vi "Create Line Seg.vi"(6 "Number of Points":i32=100, 7 "Y 2":dbl(slide) scale=0.0..10.0, 8 "X 2":dbl(slide) scale=0.0..10.0, 9 "Y 1":dbl(slide) scale=0.0..10.0, 10 "X 1":dbl(slide) scale=0.0..10.0) -> (3 "Line Segment":cluster{dbl[], dbl[]}(graph))   [LabVIEW 2013]
uses:
  <vilib>/Analysis/NI_AALPro.lvlib
panel:
  out "Plot With Point Markers":cluster{dbl[], dbl[]}[](graph)
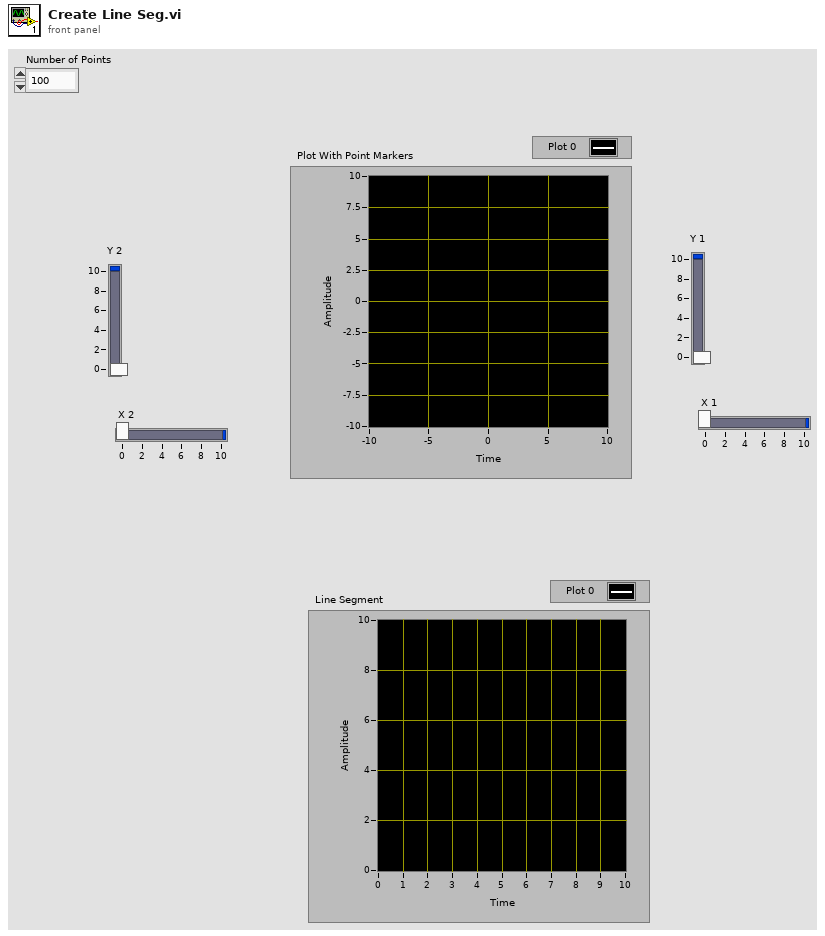
[diagram p1: front panel]
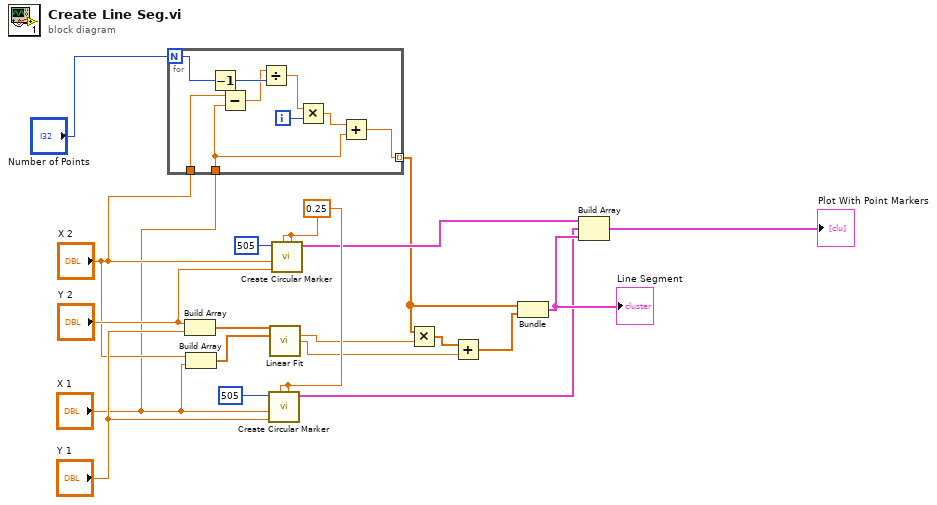
[diagram p0: block diagram]
diagram:
  w18 = 0.25 ("X Radius")
  n1 = for {
    N: "Number of Points" -> [w28]
    tunnel: [w23] -> w9 mode=indexing
    tunnel: "X 2" -> [w24]
    tunnel: "X 1" -> [w22]
    i -> [w26]
    n2 = Decrement(x=w28) -> (x-1=w21:i32)
    n3 = Subtract(x=w24, y=w22) -> (x-y=w20:dbl)
    n4 = Divide(x=w20, y=w21) -> (x/y=w27:dbl)
    n5 = Multiply(x=w27, y=w26) -> (x*y=w25:dbl)
    n6 = Add(x=w25, y=w22) -> (x+y=w23:dbl)
  }
  n7 = Build Array("Y 2", "Y 1") -> (w5:dbl[])
  n8 = Build Array("X 2", "X 1") -> (w4:dbl[])
  n9 = call "Create Circular Marker.vi"("Y Radius"=w18, "X Radius"=w18, "Y Center"="Y 1", "X Center"="X 1", "Number of Points"=505) -> ("XY Graph"=w16:cluster{dbl[], dbl[]})  [unwired: 6 in]
  n10 = call <vilib>:"Linear Fit.vi"("Y"=w5, "X"=w4) -> ("slope"=w7:dbl, "intercept"=w6:dbl)  [unwired: 9 in, 3 out]
  n11 = call "Create Circular Marker.vi"("Y Radius"=w18, "X Radius"=w18, "Y Center"="Y 2", "X Center"="X 2", "Number of Points"=505) -> ("XY Graph"=w13:cluster{dbl[], dbl[]})  [unwired: 6 in]
  n12 = Multiply(x=w9, y=w7) -> (x*y=w8:dbl[])
  n13 = Add(x=w8, y=w6) -> (x+y=w10:dbl[])
  n14 = Bundle(w9, w10) -> (w19:cluster{dbl[], dbl[]})  [unwired: 1 in]
  "Line Segment" <- w19
  n15 = Build Array(w13, w16, w19) -> (→"Plot With Point Markers":cluster{dbl[], dbl[]}[])
